vi "Raycaster_CollisionTest.vi"(5 "Map Address":u32, 6 "Y Axis (F)":bool, 7 "Other Axis Position":fxp<+/-,32,16> format="%#_21g", 8 "Forward?":bool, 9 "Speed":fxp<+/-,32,16> format="%#_21g", 10 "Position":fxp<+/-,32,16> format="%#_21g", 11 "Direction":fxp<+/-,32,16>) -> (3 "New Position":fxp<+/-,32,16>)   [LabVIEW 2020]
uses:
  Map_GetMaps.vi
  <vilib>/Utility/file.llb/Application Directory.vi
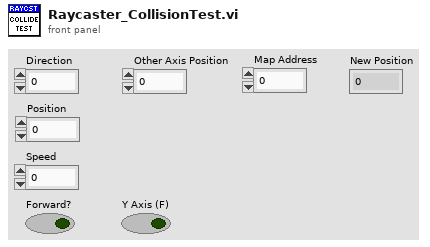
[diagram p1: front panel]
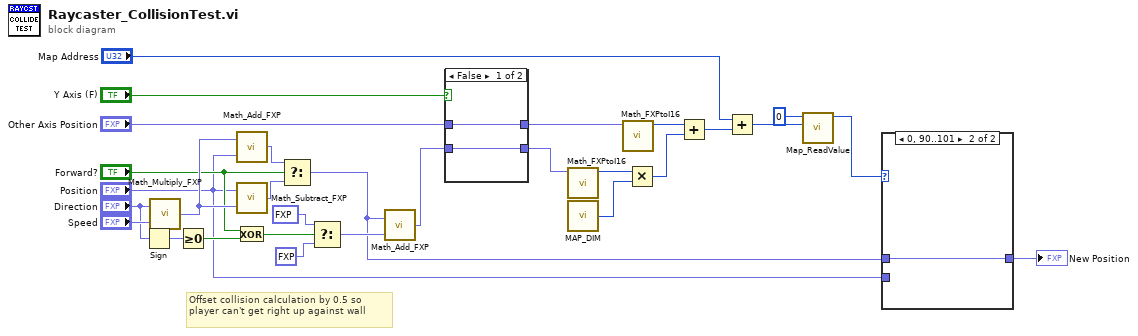
[diagram p0: block diagram]
diagram:
  # "Offset collision calculation by 0.5 so player can't get right up against wall"
  n1 = Sign(1:"Direction") -> (0:w16:fxp<+/-,2,2>)
  n2 = call "Math_Multiply_FXP.vi"("y"="Speed", "x"="Direction") -> ("x*y"=w17:fxp<+/-,32,16>)
  n3 = Greater Or Equal To 0?(x=w16) -> (x >= 0?=w9:bool)
  n4 = call "Math_Add_FXP.vi"("y"="Position", "x"=w17) -> ("x*y"=w19:fxp<+/-,32,16>)
  n5 = call "Math_Subtract_FXP.vi"("y"=w17, "x"="Position") -> ("x*y"=w18:fxp<+/-,32,16>)
  n6 = Exclusive Or(1:w9, 2:"Forward?") -> (0:w8:bool)
  n7 = Select(t=w19, s="Forward?", f=w18) -> (s? t:f=w6:fxp<+/-,32,16>)
  n8 = Select(t=fxp<+/-,32,16> -0.5 ("s? t:f"), s=w8, f=fxp<+/-,32,16> 0.5 ("s? t:f")) -> (s? t:f=w14:fxp<+/-,32,16>)
  n9 = call "Math_Add_FXP.vi"("y"=w14, "x"=w6) -> ("x*y"=w15:fxp<+/-,32,16>)
  n10 = case shown="False" "Y Axis (F)" {
    tunnel: "Other Axis Position" -> [w31 w33]
    tunnel: [w31 w32] -> w23
    tunnel: w15 -> [w30 w32]
    tunnel: [w30 w33] -> w22
    frame False {
    }
    frame True {
    }
  }
  n11 = call "Math_FXPtoI16.vi"("FXP"=w22) -> ("I16"=w28:i16)  [unwired: 10 in]
  n12 = call "MAP_DIM.vi"() -> ("MAP_DIM"=w26:i16)
  n13 = call "Math_FXPtoI16.vi"("FXP"=w23) -> ("I16"=w27:i16)  [unwired: 10 in]
  n14 = Multiply(x=w28, y=w26) -> (x*y=w29:i16)
  n15 = Add(x=w27, y=w29) -> (x+y=w3:i16)
  n16 = Add(x="Map Address", y=w3) -> (x+y=w2:u32)
  n17 = call "Map_ReadValue.vi"("Address"=w2, "Plane"=u8 0) -> ("Value"=w7:u8)  [unwired: 9 in]
  n18 = case shown="0, 90..101" w7 {
    tunnel: w6 -> [_ w35]
    tunnel: "Position" -> [w34 _]
    tunnel: [w34 w35] -> w4
    frame Default {
    }
    frame 0, 90..101 {
    }
  }
  "New Position" <- w4
